vi "Disconnect.vi"(8 "error in (no error)":errorcluster, 11 "Postgres Connector In":refnum<class "Postgres Connector.lvclass">) -> (0 "error out":errorcluster, 3 "Postgres Connector Out":refnum<class "Postgres Connector.lvclass">)   [LabVIEW 2020, in "Postgres Connector.lvclass"]
doc: "VI used at the end to close and clear the connections\ns"
uses:
  Postgres Connector.lvclass
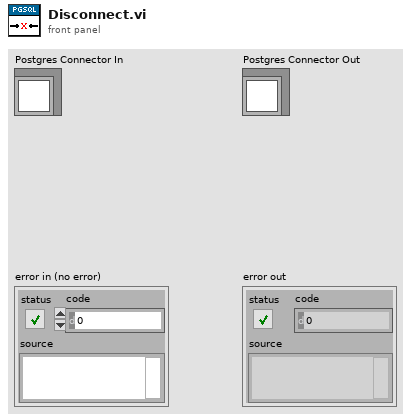
[diagram p1: front panel]
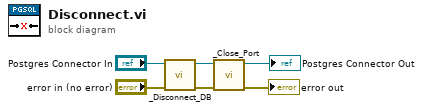
[diagram p0: block diagram]
diagram:
  n1 = call "_Disconnect_DB.vi"("error in (no error)"="error in (no error)", "Postgres Connector In"="Postgres Connector In") -> ("error out"=w2:errorcluster, "Postgres Connector Out"=w1:refnum<class "Postgres Connector.lvclass">)  [unwired: 8 in]
  n2 = call "_Close_Port.vi"("error in (no error)"=w2, "Postgres Connector.lvclass"=w1) -> ("error out"=→"error out":errorcluster, "output cluster"=→"Postgres Connector Out":refnum<class "Postgres Connector.lvclass">)  [unwired: 8 in]
